vi "9205_CV_test.vi"() -> ()   [LabVIEW 2015]
uses:
  <vilib>/Utility/sysdir.llb/System Directory Type.ctl
  <vilib>/Utility/file.llb/Write Delimited Spreadsheet (string).vi
panel:
  out "Saving 2":bool
  out "Saving":bool
  in  "number of samples":i32=1000
  in  "rate":dbl=10000.0
  in  "device name":tag="cDAQ2Mod1"
  in  "Error In":errorcluster
  out "Time":timestamp
  in  "Stop":bool
  out "tpath":path
  in  "Save Sw":bool
  out "Real-Time":dynamicdata(graph)
  out "計算結果":dynamicdata(graph)
  out "Full-save-scale":dbl[][](graph)
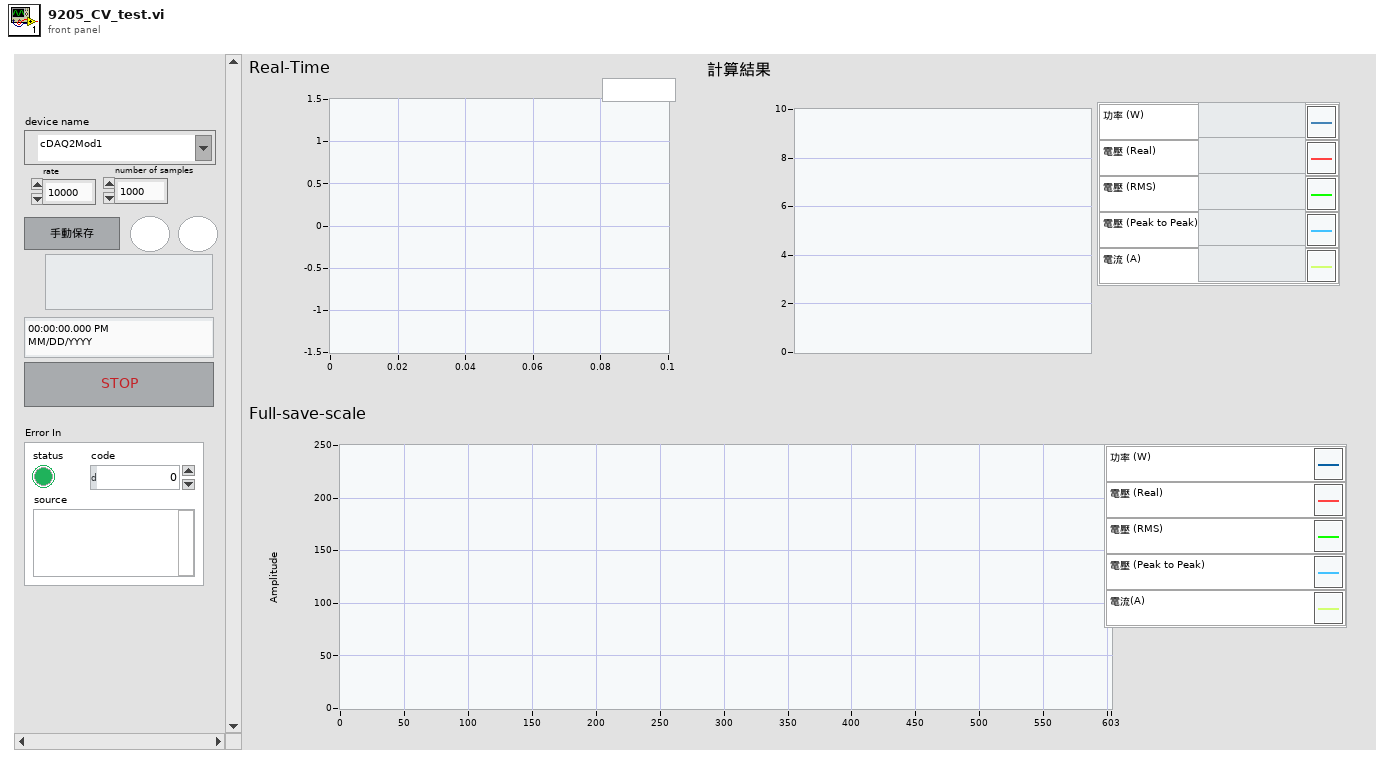
[diagram p1: front panel]
types:
  T1 = typedef "System Directory Type.ctl" = i32
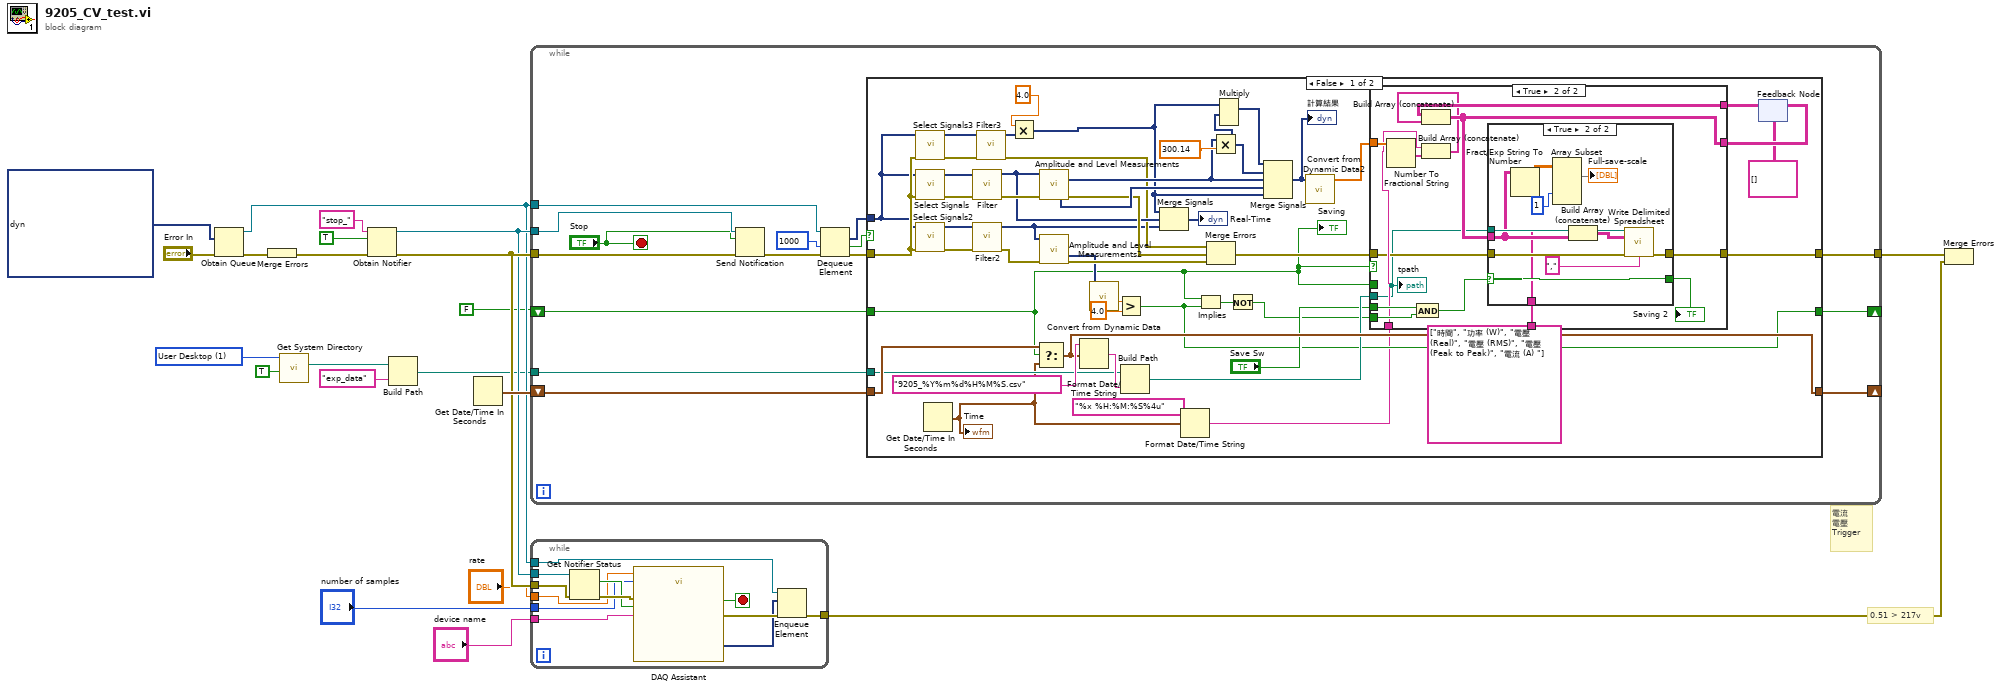
[diagram p0: block diagram]
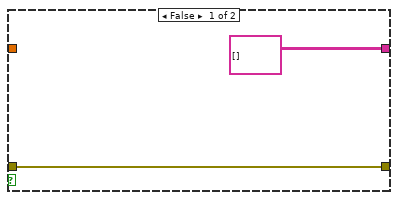
[diagram p2: hidden frame]
diagram:
  w3 = T1 1 items=["User Home"=0, "User Desktop"=1, "User Documents"=2, "User Application Data"=3, "User Preferences"=4, "User Temporary"=5, "Public Documents"=6, "Public Application Data"=7, "Public Preferences"=8, "Public Cache"=13, "System Core Libraries"=9, "System Installed Libraries"=10, "Application Files"=11, "Boot Volume Root"=12] ("system directory type")
  # "0.51 > 217v"
  # "電流\n電壓\nTrigger"
  n1 = Obtain Queue(element data type=dynamicdata [] ("data"), error in (no error)="Error In") -> (queue out=w7:refnum<queue>, error out=w21:errorcluster)  [unwired: 3 in, 1 out]
  n2 = Merge Errors(w21) -> (w19:errorcluster)
  n3 = call <vilib>:"Get System Directory.vi"("create directory if not found? (F)"=TRUE, "system directory type"=w3) -> ("system directory"=w5:path)  [unwired: 9 in]
  n4 = Obtain Notifier(name (unnamed)="stop_", notification data type=TRUE, error in (no error)=w19) -> (notifier out=w14:refnum<notifier>, error out=w15:errorcluster)  [unwired: 1 in, 1 out]
  n5 = Build Path(base path=w5, name or relative path="exp_data") -> (appended path=w2:path)
  n6 = Get Date/Time In Seconds() -> (seconds since 1Jan1904=w16:timestamp)
  n7 = while {
    tunnel: w15 -> [w36]
    tunnel: w14 -> [w35]
    tunnel: [w27] -> w8
    shift-right: [w33] -> _
    shift-left: w16 -> [w34]
    tunnel: w7 -> [w31]
    tunnel: w2 -> [w24]
    shift-right: [w22] -> _
    shift-left: FALSE -> [w23]
    stop <- "Stop" stop-if-true
    n8 = Send Notification(notification="Stop", notifier=w35, error in (no error)=w36) -> (error out=w32:errorcluster)  [unwired: 1 out]
    n9 = Dequeue Element(queue=w31, timeout in ms (-1)=1000, error in (no error)=w32) -> (element=w28:dynamicdata, timed out?=w29:bool, error out=w26:errorcluster)  [unwired: 1 out]
    n10 = case shown="False" w29 {
      tunnel: w34 -> [w84 w117]
      tunnel: [w83 w117] -> w33
      tunnel: w28 -> [w70 _]
      tunnel: [w80 w116] -> w27
      tunnel: w26 -> [w71 w116]
      tunnel: w24 -> [w81 _]
      tunnel: w23 -> [w43 w115]
      tunnel: [w42 w115] -> w22
      frame False {
        n11 = call "Select Signals3"("error in (no error)"=w71, "Signals"=w70) -> ("error out"=w59:errorcluster, "Signal Out"=w65:dynamicdata)  [unwired: 8 in]
        n12 = call "Select Signals"("error in (no error)"=w71, "Signals"=w70) -> ("error out"=w73:errorcluster, "Signal Out"=w75:dynamicdata)  [unwired: 8 in]
        n13 = call "Select Signals2"("error in (no error)"=w71, "Signals"=w70) -> ("error out"=w68:errorcluster, "Signal Out"=w67:dynamicdata)  [unwired: 8 in]
        n14 = Get Date/Time In Seconds() -> (seconds since 1Jan1904=w40:timestamp)
        "Time" <- w40
        n15 = call "Filter"("error in (no error)"=w73, "Signal"=w75) -> ("error out"=w74:errorcluster, "Filtered Signal"=w72:dynamicdata)  [unwired: 8 in]
        n16 = call "Filter2"("error in (no error)"=w68, "Signal"=w67) -> ("error out"=w58:errorcluster, "Filtered Signal"=w55:dynamicdata)  [unwired: 8 in]
        n17 = call "Filter3"("error in (no error)"=w59, "Signal"=w65) -> ("error out"=w56:errorcluster, "Filtered Signal"=w64:dynamicdata)  [unwired: 8 in]
        n18 = Multiply(x=4.0, y=w64) -> (x*y=w37:dynamicdata)
        n19 = Select(t=w84, s=w43, f=w40) -> (s? t:f=w83:timestamp)
        n20 = call "Amplitude and Level Measurements"("Signals"=w72, "error in (no error)"=w74) -> ("RMS"=w62:dynamicdata, "Peak to Peak"=w77:dynamicdata, "error out"=w76:errorcluster)  [unwired: 11 in]
        n21 = call "Amplitude and Level Measurements2"("Signals"=w55, "error in (no error)"=w58) -> ("Positive Peak"=w53:dynamicdata, "error out"=w54:errorcluster)  [unwired: 12 in]
        n22 = Format Date/Time String(time format string (%c)="9205_%Y%m%d%H%M%S.csv", seconds (now)=w83) -> (date/time string=w82:string)  [unwired: 1 in]
        n23 = call "Convert from Dynamic Data"("Dynamic Data Type"=w53) -> ("Scalar"=w51:dbl)  [unwired: 3 in]
        n24 = Greater?(x=w51, y=4.0) -> (0:w42:bool)
        n25 = Build Path(base path=w81, name or relative path=w82) -> (appended path=w79:path)
        n26 = Merge Signals(w37, w72, w55) -> (→"Real-Time":dynamicdata)
        n27 = Format Date/Time String(time format string (%c)="%x %H:%M:%S%4u", seconds (now)=w40) -> (date/time string=w39:string)  [unwired: 1 in]
        n28 = Implies(1:w42, 2:w43) -> (0:w45:bool)
        n29 = Merge Errors(w56, w76, w54) -> (w57:errorcluster)
        n30 = Multiply(x=w62, y=300.14) -> (x*y=w61:dynamicdata)
        n31 = Multiply(1:w61, 2:w37) -> (0:w60:dynamicdata)  [unwired: 1 in, 1 out]
        n32 = Not(x=w45) -> (.not. x?=w44:bool)
        n33 = Merge Signals(w60, w61, w62, w77, w37) -> (w50:dynamicdata)
        "計算結果" <- w50
        n34 = call "Convert from Dynamic Data2"("Dynamic Data Type"=w50) -> ("Array"=w49:dbl[])  [unwired: 3 in]
        n35 = feedback #1(string[][] []) -> (w47:string[][])
        n36 = case shown="True" w43 {
          tunnel: w43 -> [_ _]
          tunnel: w57 -> [w87 w93]
          tunnel: [w87 w92] -> w80
          tunnel: w79 -> [_ w91]
          tunnel: "Save Sw" -> [_ w101]
          tunnel: w49 -> [_ w98]
          tunnel: [string[][] [] w99] -> w48
          tunnel: w47 -> [_ w97]
          tunnel: w44 -> [_ w100]
          tunnel: w39 -> [_ w95]
          tunnel: string[] ["時間", "功率 (W)", "電壓 (Real)", "電壓 (RMS)", "電壓 (Peak to Peak)", "電流 (A) "] ("array") -> [_ w88]
          frame False {
          }
          frame True {
            n37 = Number To Fractional String(number=w98) -> (F-format string=w96:string[])  [unwired: 3 in]
            n38 = And(x=w101, y=w100) -> (x .and. y?=w90:bool)
            n39 = Build Array (concatenate)(w95, w96) -> (w94:string[])
            n40 = Build Array (concatenate)(w97, w94) -> (w99:string[][])
            n41 = case shown="True" w90 {
              selector: w90 -> [w103 w110]
              tunnel: w93 -> [w102 w114]
              tunnel: [w102 w113] -> w92
              tunnel: w91 -> [_ w112]
              tunnel: w99 -> [_ w109]
              tunnel: [w103 w110] -> w89
              tunnel: w88 -> [_ w104]
              frame False {
              }
              frame True {
                n42 = Fract/Exp String To Number(string=w109) -> (number=w108:dbl[][])  [unwired: 3 in, 1 out]
                n43 = Array Subset(array=w108, index (col)=1 ("index")) -> (→"Full-save-scale":dbl[][])  [unwired: 3 in]
                n44 = Build Array (concatenate)(w104, w109) -> (w105:string[][])
                n45 = call-poly <vilib>:"Write Delimited Spreadsheet.vi"("file path (dialog if empty)"=w112, "2D data"=w105, "error in (no error)"=w114, "delimiter (\\t)"="," ("delimiter (\\t)")) -> ("error out"=w113:errorcluster)  [unwired: 10 in, 1 out]
              }
            }
            "Saving 2" <- w89
            "tpath" <- w91
          }
        }
        n46 = feedback-in #1(w48) -> ()
        "Saving" <- w43
      }
      frame True {
      }
    }
  }
  n47 = while {
    tunnel: w7 -> [w128]
    tunnel: w15 -> [w125]
    tunnel: w14 -> [w124]
    tunnel: "number of samples" -> [w122]
    tunnel: "rate" -> [w121]
    tunnel: "device name" -> [w120]
    tunnel: [w118] -> w9
    stop <- w129 stop-if-true
    n48 = Get Notifier Status(notifier=w124, error in (no error)=w125) -> (current notification=w123:bool, error out=w126:errorcluster)  [unwired: 3 out]
    n49 = call "DAQ Assistant"("rate"=w121, "number of samples"=w122, "error in"=w126, "stop (F)"=w123, "device name"=w120) -> ("data"=w119:dynamicdata, "stopped"=w129:bool, "error out"=w127:errorcluster)  [unwired: 11 in, 1 out]
    n50 = Enqueue Element(queue=w128, element=w119, error in (no error)=w127) -> (error out=w118:errorcluster)  [unwired: 1 in, 2 out]
  }
  n51 = Merge Errors(w8, w9) -> ()  [unwired: 1 out]
